vi "SelectedGoalCrosshair.vi"(10 "SelectedGoalSubarray":dbl[](array[numeric]), 11 "Image In":T1) -> (3 "Image Out":T1)   [LabVIEW 2012]
uses:
  <vilib>/vision/Image Controls.llb/IMAQ Image.ctl
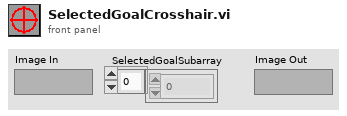
[diagram p1: front panel]
types:
  T1 = typedef "IMAQ Image.ctl" = refnum<image>
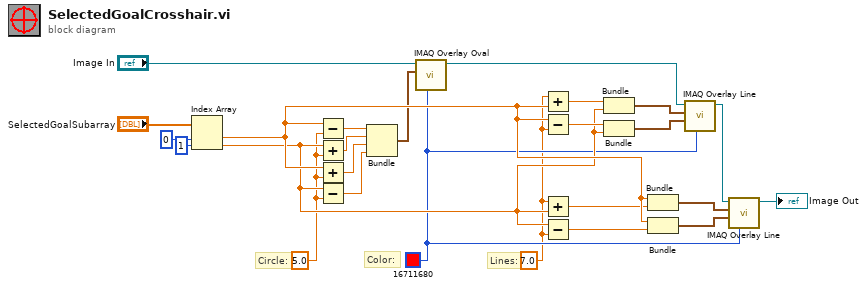
[diagram p0: block diagram]
diagram:
  w4 = u32 16711680 ("Color")
  w3 = 7.0 ("x")
  w6 = 5.0 ("y")
  # "Color:"
  # "Lines:"
  # "Circle:"
  n1 = Index Array(array="SelectedGoalSubarray", index #1=0 ("index"), index #2=1 ("index")) -> (element #1=w25:dbl, element #2=w7:dbl)
  n2 = Subtract(x=w25, y=w6) -> (x-y=w20:dbl)
  n3 = Add(x=w7, y=w6) -> (x+y=w21:dbl)
  n4 = Add(x=w25, y=w6) -> (x+y=w19:dbl)
  n5 = Subtract(x=w7, y=w6) -> (x-y=w5:dbl)
  n6 = Bundle(w20, w21, w19, w5) -> (w18:cluster{dbl, dbl, dbl, dbl})  [unwired: 1 in]
  n7 = call "IMAQ Overlay Oval"("Color"=w4, "Bounding Rectangle"=w18, "Image"="Image In") -> ("Image Out"=w8:T1)  [unwired: 7 in, 1 out]
  n8 = Add(x=w3, y=w25) -> (x+y=w16:dbl)
  n9 = Subtract(x=w25, y=w3) -> (x-y=w17:dbl)
  n10 = Add(x=w3, y=w7) -> (x+y=w11:dbl)
  n11 = Subtract(x=w7, y=w3) -> (x-y=w10:dbl)
  n12 = Bundle(w16, "Numeric"=w7) -> (w15:cluster{dbl, "Numeric":dbl})  [unwired: 1 in]
  n13 = Bundle(w17, "Numeric"=w7) -> (w14:cluster{dbl, "Numeric":dbl})  [unwired: 1 in]
  n14 = Bundle("Numeric"=w25, w11) -> (w13:cluster{"Numeric":dbl, dbl})  [unwired: 1 in]
  n15 = Bundle("Numeric"=w25, w10) -> (w12:cluster{"Numeric":dbl, dbl})  [unwired: 1 in]
  n16 = call "IMAQ Overlay Line"("Color"=w4, "End Point"=w14, "Start Point"=w15, "Image"=w8) -> ("Image Out"=w9:T1)  [unwired: 6 in, 1 out]
  n17 = call "IMAQ Overlay Line"("Color"=w4, "End Point"=w12, "Start Point"=w13, "Image"=w9) -> ("Image Out"=→"Image Out":T1)  [unwired: 6 in, 1 out]
